vi "getRDfilepath.vi"(9 "templatePath":path, 10 "rowIndex":i32, 11 "Result files to read":path[](array[path])) -> (1 "selectedRowNum":i32, 2 "rawDataPath":path, 3 "Results file":path)   [LabVIEW 2021]
uses:
  Anemometry/Anemometry Sub Vis/Data_plotting_vis/Results_plotter_Global.vi
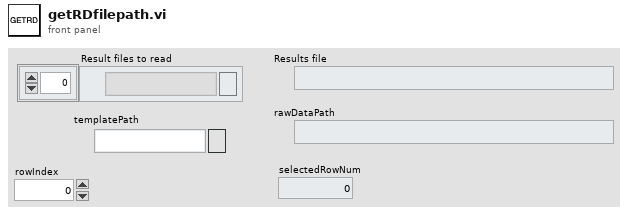
[diagram p1: front panel]
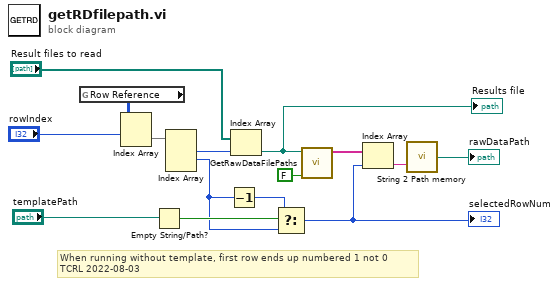
[diagram p0: block diagram]
diagram:
  # "When running without template, first row ends up numbered 1 not 0\nTCRL 2022-08-03"
  n1 = global read "Results_plotter_Global.vi" "Row Reference"() -> (w7:i32[][])
  n2 = Index Array(array=w7, index (row)="rowIndex") -> (element=w11:i32[])  [unwired: 1 in]
  n3 = Empty String/Path?(string/path="templatePath") -> (empty?=w6:bool)
  n4 = Index Array(array=w11) -> (element #1=w10:i32, element #2=w5:i32)  [unwired: 3 in, 1 out]
  n5 = Decrement(x=w5) -> (x-1=w3:i32)
  n6 = Index Array(array="Result files to read", index=w10) -> (element=w12:path)
  "Results file" <- w12
  n7 = Select(t=w3, s=w6, f=w5) -> (s? t:f=w4:i32)
  "selectedRowNum" <- w4
  n8 = call "GetRawDataFilePaths.vi"("Force Fresh File Read?"=FALSE ("Fresh File Read?"), "Results file or Folder"=w12) -> ("RawDataFilePaths"=w13:string[])  [unwired: 9 in]
  n9 = Index Array(array=w13, index=w4) -> (element=w14:string)
  n10 = call "String 2 Path memory.vi"("Input String"=w14) -> ("path"=→"rawDataPath":path)  [unwired: 1 in]
